vi "CIF Template UI.vi"() -> ()   [LabVIEW 2021, in "CIF Template UI.lvlib"]
uses:
  CIF Template UI.lvlib
  <vilib>/CIF Foundation/CIF Core/CIFUI/Typedef/Run Listen Button.ctl
  <vilib>/CIF Foundation/CIF Core/CIFUI/Typedef/Core UI References.ctl
  <vilib>/CIF Foundation/CIF Core/CIFUI/CIF_UI.lvclass/CIF_UI.ctl
  <vilib>/CIF Foundation/CIF Core/CIFUI/Utilities/Get Human Readable Error.vi
  <vilib>/CIF Foundation/CIF Utilities/Errors/Append Error Location.vi
  <vilib>/CIF Foundation/CIF Core/CIFUI/UI Element Update/Empty Tree by Reference.vi
  <vilib>/CIF Foundation/CIF Core/CIFUI/UI Element Update/Empty Table by Reference.vi
  <vilib>/CIF Foundation/CIF Core/CIFUI/UI Element Update/Initialize Manager Tab by Reference.vi
  <vilib>/CIF Foundation/CIF Utilities/Errors/Human Readable Error Message.vi
  <vilib>/CIF Foundation/CIF Core/CIFUI/CIF_UI.lvclass
  Grpc/Template_wrapper/Template_Wrapper.lvlib
  <vilib>/Utility/LVLibp/NI_PackedLibraryUtility.lvlib
panel:
  in  "Session Id":u64
  in  "EXIT":bool
  in  "Address with Port":string="192.168.1.160:12345"
  in  "Clear Local Error":bool
  out "Connected":bool
  in  "Unload":bool
  in  "Refresh Button":bool
  in  "Run Listen":T1
  in  "Connection":bool
  out "Local Error":string
  in  "Plugin Status":string[][](table)
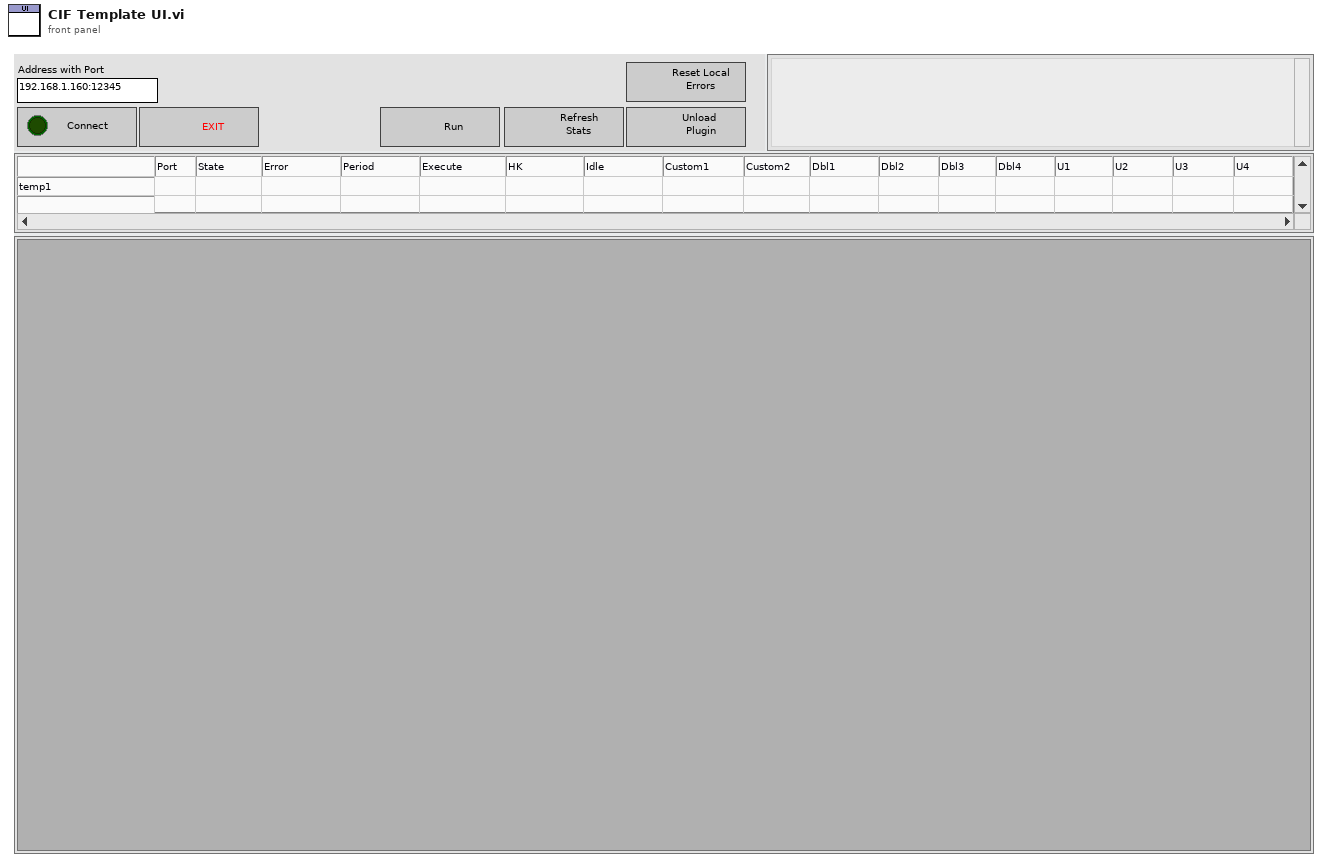
[diagram p1: front panel]
types:
  T1 = typedef "CIF_UI.lvclass/Run Listen Button.ctl" = bool
  T2 = typedef "CIF_UI.lvclass/Core UI References.ctl" = cluster{"Discovered Plugins":refnum<vi>, "Discovered Plugins Valid":bool, "Loaded Plugins":refnum<vi>, "Loaded Plugins Valid":bool, "Publisher Channels":refnum<vi>, "Publisher Channels Valid":bool, "Subscriber Channels":refnum<vi>, "Subscriber Channels Valid":bool, "Plugin Status":refnum<vi>, "Plugin Status Valid":bool, "Channel Connection":refnum<vi>, "Channel Connection Valid":bool, "New Plugin Load":refnum<vi>, "New Plugin Load Valid":bool, "Errors":refnum<vi>, "Errors Valid":bool, "Plugin to Abort":refnum<vi>, "Plugin to Abort Valid":bool, "Connection":refnum<vi>, "Connection Valid":bool, "Exit":refnum<vi>, "Exit Valid":bool, "Run Listen":refnum<vi>, "Run Listen Valid":bool, "CIF Manager Tab":refnum<vi>, "Manger Tab Valid":bool, "Clear Local Error":refnum<vi>, "Clear Local Error Valid":bool, "Local Error":refnum<vi>, "Local Error Valid":bool, "System Errors":refnum<vi>, "System Errors Valid":bool, "Plugin Selection":refnum<vi>, "Plugin Selection Valid":bool}
  T3 = typedef "CIF_InstrumentStudio Plugin SDK.lvlib/Event Registration Refnum.ctl" = refnum<event-registration>
  T4 = cluster{"Event Refnum":T3, "Event Registration Refnum":refnum<event-registration>}
  T5 = typedef "grpc-lvsupport-release.lvlib/grpcId.ctl" = u64
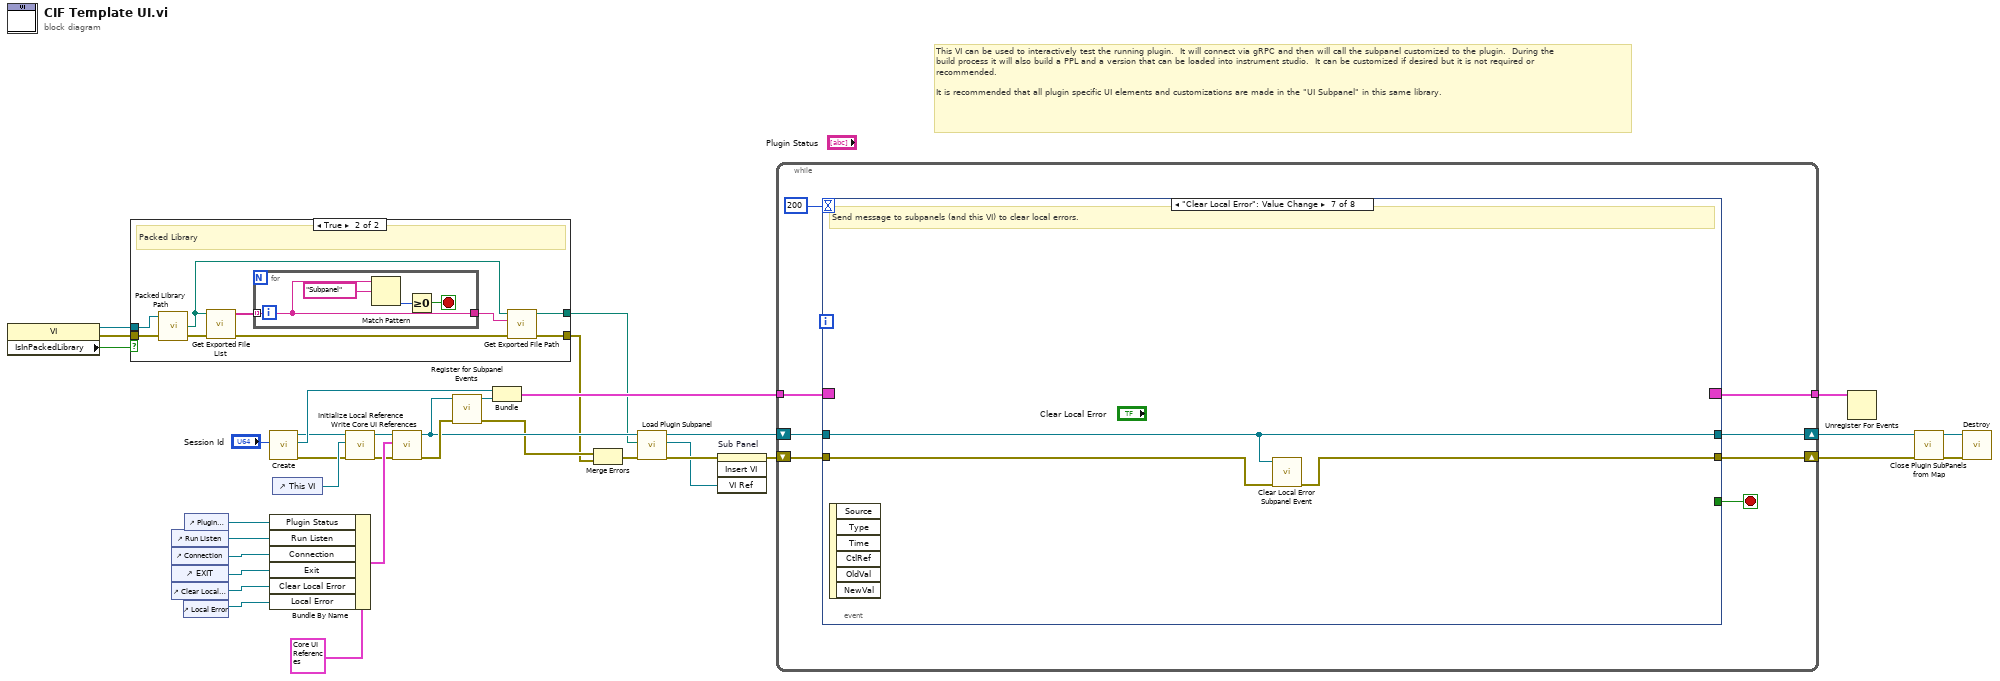
[diagram p0: block diagram]
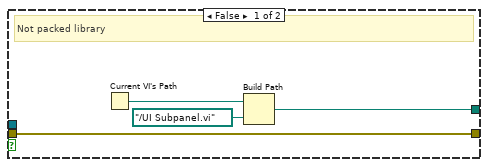
[diagram p2: hidden frame]
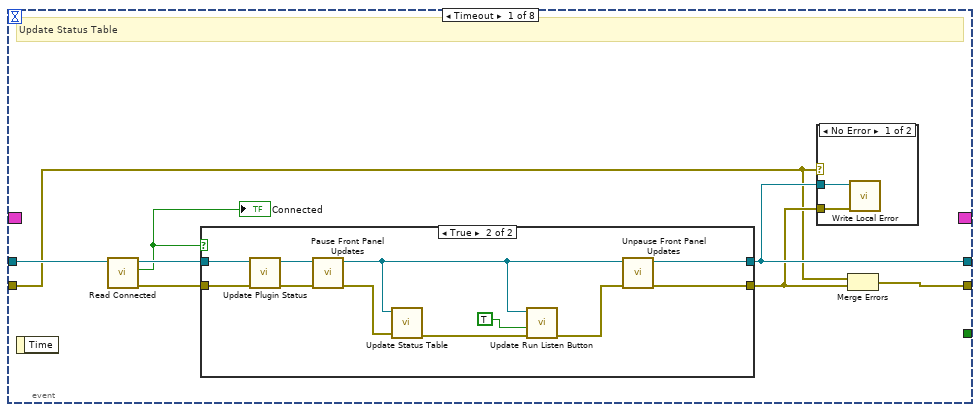
[diagram p3: hidden frame]
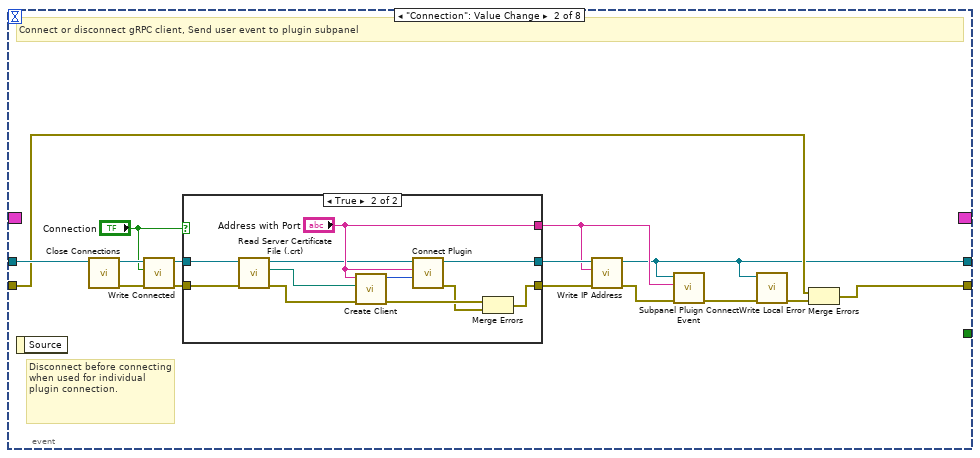
[diagram p6: hidden frame]
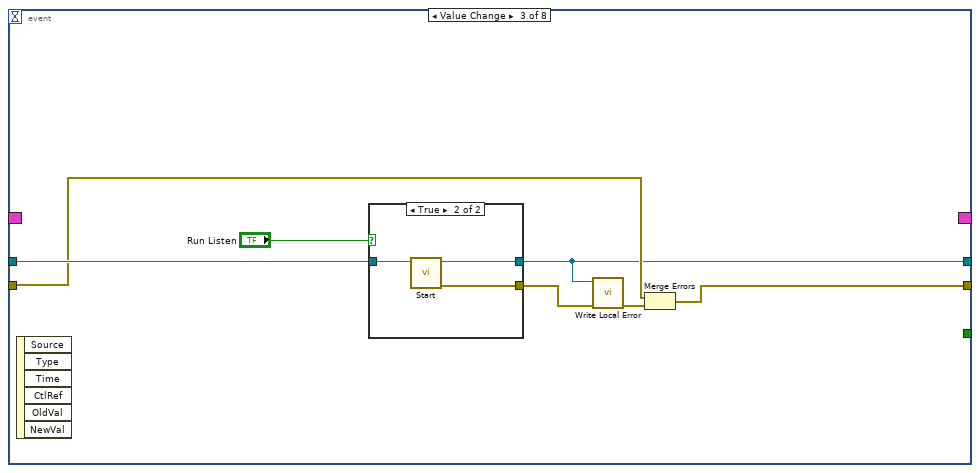
[diagram p8: hidden frame]
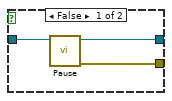
[diagram p9: hidden frame]
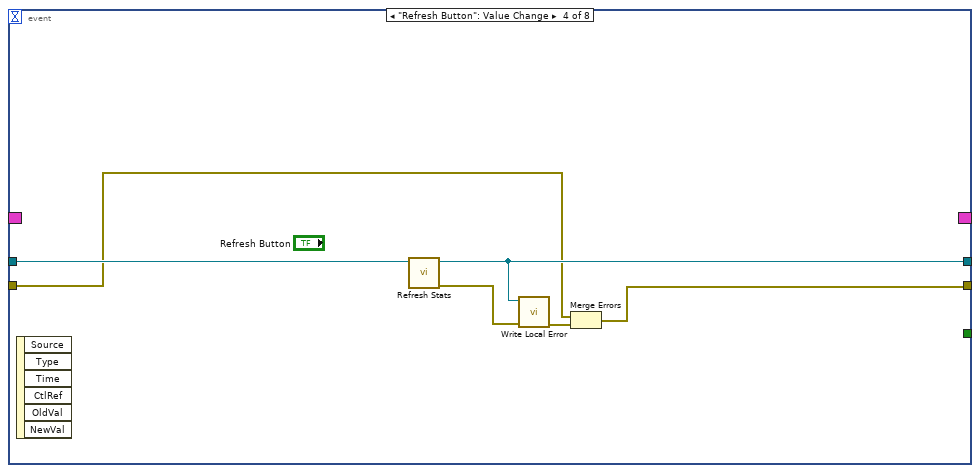
[diagram p10: hidden frame]
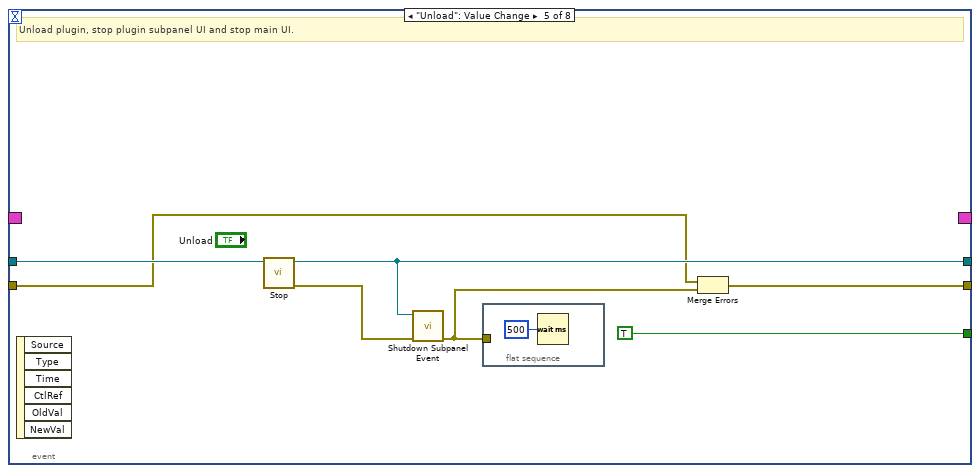
[diagram p11: hidden frame]
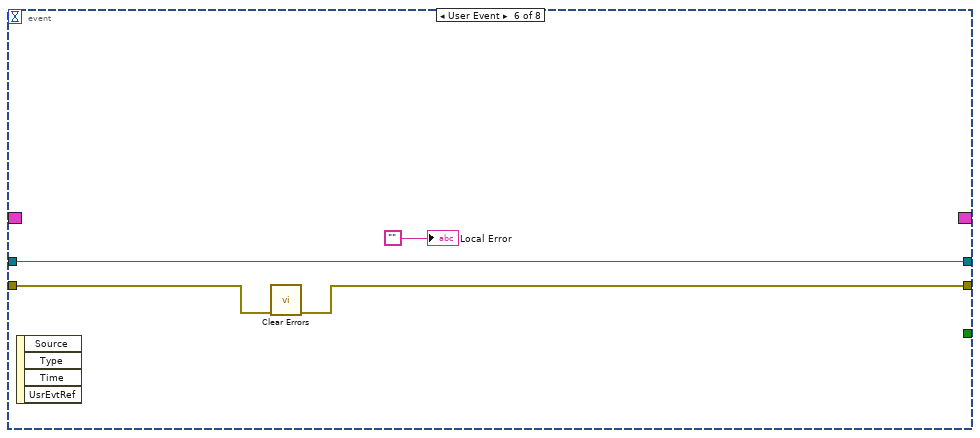
[diagram p12: hidden frame]
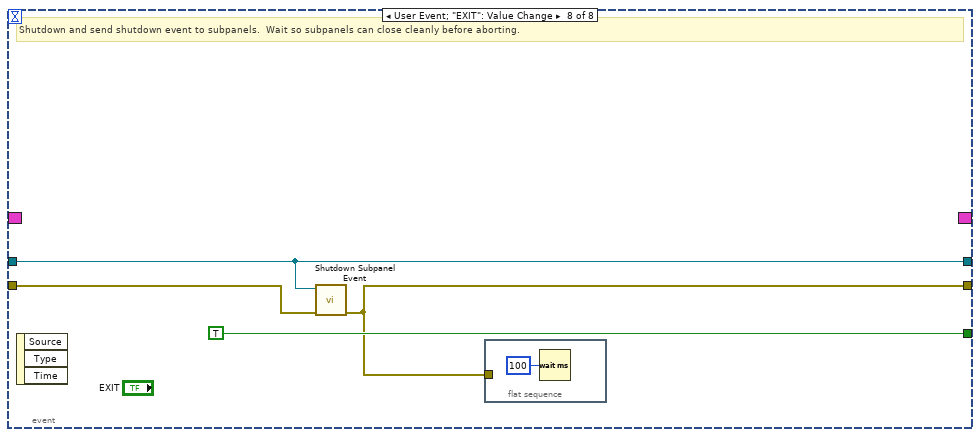
[diagram p13: hidden frame]
diagram:
  # "This VI can be used to interactively test the running plugin.  It will connect via gRPC and then will call the subpanel customized to the plugin.  During the build process it will also build a PPL and a version that can be loaded into instrument studio.  It can be customized if desired but it is not required or recommended.  \n\nIt is recommended that all plugin specific UI elements and customizations are made in the \"UI Subpanel\" in this same library."
  n1 = property class="VI"() -> (reference out=w8:refnum<vi>, error out=w7:errorcluster, "IsInPackedLibrary"=w9:bool)  [unwired: 2 in]
  n2 = case shown="True" w9 {
    tunnel: w8 -> [_ w48]
    tunnel: w7 -> [w36 w47]
    tunnel: [w39 w41] -> w6
    tunnel: [w36 w40] -> w3
    frame False {
      # "Not packed library"
      n3 = Current VI's Path() -> (path=w38:path)
      n4 = Build Path(base path=w38, name or relative path=path "../UI Subpanel.vi" ("Path")) -> (appended path=w39:path)
    }
    frame True {
      # "Packed Library"
      n5 = call <vilib>:"Packed Library Path.vi"("error in (no error)"=w47, "vi reference"=w48) -> ("error out"=w42:errorcluster, "packed library path"=w43:path)  [unwired: 1 in, 1 out]
      n6 = call <vilib>:"Get Exported File List.vi"("error in (no error)"=w42, "packed library path"=w43) -> ("error out"=w45:errorcluster, "qualified names"=w44:string[])  [unwired: 7 in, 1 out]
      n7 = for {
        tunnel: w44 -> [w49] mode=indexing
        tunnel: [w49] -> w46
        stop <- w51 stop-if-true
        n8 = Match Pattern(string=w49, regular expression="Subpanel") -> (offset past match=w52:i32)  [unwired: 1 in, 3 out]
        n9 = Greater Or Equal To 0?(x=w52) -> (x >= 0?=w51:bool)
      }
      n10 = call <vilib>:"Get Exported File Path.vi"("error in (no error)"=w45, "qualified name"=w46, "packed library path"=w43) -> ("error out"=w40:errorcluster, "path"=w41:path)  [unwired: 7 in]
    }
  }
  n11 = control-ref of="Run Listen"() -> (w29:refnum<vi>)
  n12 = control-ref of="Connection"() -> (w26:refnum<vi>)
  n13 = control-ref of="EXIT"() -> (w25:refnum<vi>)
  n14 = control-ref of="Clear Local Error"() -> (w24:refnum<vi>)
  n15 = control-ref of="Local Error"() -> (w23:refnum<vi>)
  n16 = control-ref of="Plugin Status"() -> (w33:refnum<vi>)
  n17 = call <vilib>:"Create.vi"("Session Id"="Session Id") -> ("error out"=w20:errorcluster, "Event Refnum"=w27:T3, "CIF_UI out"=w21:refnum<class "CIF_UI.lvclass">)  [unwired: 8 in]
  n18 = Bundle By Name(cluster=T2 {"Discovered Plugins"=refnum, "Discovered Plugins Valid"=FALSE, "Loaded Plugins"=refnum, "Loaded Plugins Valid"=FALSE, "Publisher Channels"=refnum, "Publisher Channels Valid"=FALSE, "Subscriber Channels"=refnum, "Subscriber Channels Valid"=FALSE, "Plugin Status"=refnum, "Plugin Status Valid"=FALSE, "Channel Connection"=refnum, "Channel Connection Valid"=FALSE, "New Plugin Load"=refnum, "New Plugin Load Valid"=FALSE, "Errors"=refnum, "Errors Valid"=FALSE, "Plugin to Abort"=refnum, "Plugin to Abort Valid"=FALSE, "Connection"=refnum, "Connection Valid"=FALSE, "Exit"=refnum, "Exit Valid"=FALSE, "Run Listen"=refnum, "Run Listen Valid"=FALSE, "CIF Manager Tab"=refnum, "Manger Tab Valid"=FALSE, "Clear Local Error"=refnum, "Clear Local Error Valid"=FALSE, "Local Error"=refnum, "Local Error Valid"=FALSE, "System Errors"=refnum, "System Errors Valid"=FALSE, "Plugin Selection"=refnum, "Plugin Selection Valid"=FALSE} ("UI References"), "Plugin Status"=w33, "Run Listen"=w29, "Connection"=w26, "Exit"=w25, "Clear Local Error"=w24, "Local Error"=w23) -> (w34:T2)
  n19 = control-ref of="This VI"() -> (w32:refnum<vi>)
  n20 = call <vilib>:"Initialize Local Reference.vi"("error in (no error)"=w20, "This VI"=w32, "CIF_UI in"=w21) -> ("error out"=w30:errorcluster, "CIF_UI out"=w31:refnum<class "CIF_UI.lvclass">)  [unwired: 7 in]
  n21 = call <vilib>:"Write Core UI References.vi"("error in (no error)"=w30, "UI References"=w34, "CIF_UI in"=w31) -> ("error out"=w19:errorcluster, "CIF_UI out"=w17:refnum<class "CIF_UI.lvclass">)  [unwired: 7 in]
  n22 = call <vilib>:"Register for Subpanel Events.vi"("error in (no error)"=w19, "CIF_UI in"=w17) -> ("error out"=w5:errorcluster, "Event Registration Refnum"=w28:refnum<event-registration>)  [unwired: 8 in]
  n23 = Bundle("Event Refnum"=w27, "Event Registration Refnum"=w28) -> (w22:T4)  [unwired: 1 in]
  n24 = Merge Errors(w5, w3) -> (w4:errorcluster)
  n25 = call <vilib>:"Load Plugin Subpanel.vi"("error in (no error)"=w4, "Path"=w6, "CIF_UI in"=w17) -> ("error out"=w15:errorcluster, "VI Reference"=w13:refnum<vi>, "CIF_UI out"=w16:refnum<class "CIF_UI.lvclass">)  [unwired: 6 in]
  n26 = invoke on="Sub Panel" class="SubPnl" method="Insert VI"(error in=w15, "VI Ref"=w13) -> (error out=w14:errorcluster)  [unwired: 2 in, 3 out]
  n27 = while {
    shift-right: [w55] -> w12
    shift-left: w16 -> [w58]
    shift-right: [w56] -> w1
    shift-left: w14 -> [w57]
    tunnel: w22 -> [w54]
    tunnel: [w53] -> w18
    stop <- w59 stop-if-true
    n28 = event shown="[6] \"Clear Local Error\": Value Change" {
      selector: w54 -> [_ _ _ _ _ _ _ _]
      dyn-events: [_ _ _ _ _ _ _ _] -> w53
      timeout: 200 -> [_ _ _ _ _ _ _ _]
      tunnel: [_ _ _ _ TRUE _ _ TRUE] -> w59
      tunnel: w58 -> [w66 w98 w118 w130 w137 w140 w143 w148]
      tunnel: w57 -> [w61 w86 w114 w125 w132 w142 w145 w147]
      tunnel: [w64 w85 w113 w126 w131 w141 w144 w146] -> w56
      tunnel: [w63 w84 w112 w127 w135 w140 w143 w148] -> w55
      event Timeout {
        # "Update Status Table"
        n29 = event-data() -> ()  [unwired: 1 in, 1 out]
        n30 = call <vilib>:"Read Connected.vi"("CIF_UI in"=w66) -> ("error out"=w67:errorcluster, "Connected"=w65:bool, "CIF_UI out"=w68:refnum<class "CIF_UI.lvclass">)  [unwired: 8 in]
        "Connected" <- w65
        n31 = case shown="True" w65 {
          tunnel: w67 -> [w71 w81]
          tunnel: [w71 w83] -> w62
          tunnel: w68 -> [w72 w80]
          tunnel: [w72 w82] -> w63
          frame False {
          }
          frame True {
            n32 = call <vilib>:"Update Plugin Status.vi"("error in (no error)"=w81, "CIF_UI in"=w80) -> ("error out"=w77:errorcluster, "CIF_UI out"=w79:refnum<class "CIF_UI.lvclass">)  [unwired: 8 in]
            n33 = call <vilib>:"Pause Front Panel Updates.vi"("error in (no error)"=w77, "CIF_UI in"=w79) -> ("error out"=w78:errorcluster, "CIF_UI out"=w74:refnum<class "CIF_UI.lvclass">)  [unwired: 8 in]
            n34 = call <vilib>:"Update Status Table.vi"("error in (no error)"=w78, "CIFManager_UI in"=w74) -> ("error out"=w76:errorcluster)  [unwired: 9 in]
            n35 = call <vilib>:"Update Run Listen Button.vi"("error in (no error)"=w76, "Use First Entry"=TRUE, "CIFManager_UI in"=w74) -> ("error out"=w75:errorcluster)  [unwired: 8 in]
            n36 = call <vilib>:"Unpause Front Panel Updates.vi"("error in (no error)"=w75, "CIF_UI in"=w74) -> ("error out"=w83:errorcluster, "CIF_UI out"=w82:refnum<class "CIF_UI.lvclass">)  [unwired: 8 in]
          }
        }
        n37 = case shown="No Error" w61 {
          tunnel: w62 -> [w70 _]
          tunnel: w63 -> [w69 _]
          frame No Error {
            n38 = call <vilib>:"Write Local Error.vi"("error in (no error)"=w70, "CIF_UI in"=w69) -> ()  [unwired: 9 in, 1 out]
          }
          frame Error {
          }
        }
        n39 = Merge Errors(w61, w62) -> (w64:errorcluster)
      }
      event "Connection": Value Change {
        # "Disconnect before connecting when used for individual plugin connection."
        # "Connect or disconnect gRPC client, Send user event to plugin subpanel"
        n40 = event-data() -> ()  [unwired: 1 in, 1 out]
        n41 = call <vilib>:"Close Connections.vi"("CIF_UI in"=w98) -> ("error out"=w96:errorcluster, "CIF_UI out"=w97:refnum<class "CIF_UI.lvclass">)  [unwired: 9 in]
        n42 = call <vilib>:"Write Connected.vi"("error in (no error)"=w96, "Connected"="Connection", "CIF_UI in"=w97) -> ("error out"=w93:errorcluster, "CIF_UI out"=w95:refnum<class "CIF_UI.lvclass">)  [unwired: 7 in]
        n43 = case shown="True" "Connection" {
          tunnel: [w100 w107] -> w92
          tunnel: [w99 w111] -> w91
          tunnel: w93 -> [w99 w104]
          tunnel: w95 -> [w100 w105]
          tunnel: [_ "Address with Port"] -> w89
          frame False {
          }
          frame True {
            n44 = call <vilib>:"Read Server Certificate File (.crt).vi"("error in (no error)"=w104, "CIF_UI in"=w105) -> ("error out"=w103:errorcluster, "Server Certificate File (.crt)"=w102:path, "CIF_UI out"=w101:refnum<class "CIF_UI.lvclass">)  [unwired: 7 in]
            n45 = call "Create Client.vi"("error in"=w103, "Server Certificate File (.crt)"=w102, "address"="Address with Port") -> ("error out"=w109:errorcluster, "gRPC ID Out"=w110:T5)  [unwired: 7 in]
            n46 = call <vilib>:"Connect Plugin.vi"("gRPC ID"=w110, "Address"="Address with Port", "CIF_UI in"=w101) -> ("error out"=w108:errorcluster, "CIF_UI out"=w107:refnum<class "CIF_UI.lvclass">)  [unwired: 7 in]
            n47 = Merge Errors(w109, w108) -> (w111:errorcluster)
          }
        }
        n48 = call <vilib>:"Write IP Address.vi"("error in (no error)"=w91, "IP Address"=w89, "CIF_UI in"=w92) -> ("error out"=w90:errorcluster, "CIF_UI out"=w84:refnum<class "CIF_UI.lvclass">)  [unwired: 7 in]
        n49 = call <vilib>:"Subpanel Pluign Connect Event.vi"("error in (no error)"=w90, "Address and Port"=w89, "CIF_UI in"=w84) -> ("error out"=w87:errorcluster)  [unwired: 8 in]
        n50 = call <vilib>:"Write Local Error.vi"("error in (no error)"=w87, "CIF_UI in"=w84) -> ("error out"=w88:errorcluster)  [unwired: 9 in]
        n51 = Merge Errors(w86, w88) -> (w85:errorcluster)
      }
      event Value Change {
        n52 = event-data() -> ()  [unwired: 1 in, 6 out]
        n53 = case shown="True" "Run Listen" {
          tunnel: w118 -> [w121 w124]
          tunnel: [w119 w123] -> w112
          tunnel: [w120 w122] -> w115
          frame False {
            n54 = call <vilib>:"Pause.vi"("CIF_Plugin_UI in"=w121) -> ("error out"=w120:errorcluster, "CIF_Plugin_UI out"=w119:refnum<class "CIF_UI.lvclass">)  [unwired: 8 in, 1 out]
          }
          frame True {
            n55 = call <vilib>:"Start.vi"("CIF_Plugin_UI in"=w124) -> ("error out"=w122:errorcluster, "CIF_Plugin_UI out"=w123:refnum<class "CIF_UI.lvclass">)  [unwired: 8 in, 1 out]
          }
        }
        n56 = call <vilib>:"Write Local Error.vi"("error in (no error)"=w115, "CIF_UI in"=w112) -> ("error out"=w116:errorcluster)  [unwired: 9 in]
        n57 = Merge Errors(w114, w116) -> (w113:errorcluster)
      }
      event "Refresh Button": Value Change {
        n58 = event-data() -> ()  [unwired: 1 in, 6 out]
        n59 = call <vilib>:"Refresh Stats.vi"("CIF_Plugin_UI in"=w130) -> ("error out"=w128:errorcluster, "CIF_Plugin_UI out"=w127:refnum<class "CIF_UI.lvclass">)  [unwired: 8 in, 1 out]
        n60 = call <vilib>:"Write Local Error.vi"("error in (no error)"=w128, "CIF_UI in"=w127) -> ("error out"=w129:errorcluster)  [unwired: 9 in]
        n61 = Merge Errors(w125, w129) -> (w126:errorcluster)
      }
      event "Unload": Value Change {
        # "Unload plugin, stop plugin subpanel UI and stop main UI."
        n62 = event-data() -> ()  [unwired: 1 in, 6 out]
        n63 = call <vilib>:"Stop.vi"("CIF_Plugin_UI in"=w137) -> ("error out"=w136:errorcluster, "CIF_Plugin_UI out"=w135:refnum<class "CIF_UI.lvclass">)  [unwired: 8 in, 1 out]
        n64 = call <vilib>:"Shutdown Subpanel Event.vi"("error in (no error)"=w136, "CIF_UI in"=w135) -> ("error out"=w133:errorcluster)  [unwired: 9 in]
        n65 = flat-sequence {
          tunnel: w133 -> [_]
          frame #0 {
            n66 = Wait (ms)(milliseconds to wait=u32 500) -> ()  [unwired: 1 out]
          }
        }
        n67 = Merge Errors(w132, w133) -> (w131:errorcluster)
      }
      event User Event {
        n68 = event-data() -> ()  [unwired: 1 in, 4 out]
        n69 = call <vilib>:"Clear Errors.vi"("error in (no error)"=w142) -> ("error out"=w141:errorcluster)  [unwired: 5 in, 1 out]
        "Local Error" <- ""
      }
      event "Clear Local Error": Value Change {
        # "Send message to subpanels (and this VI) to clear local errors."
        n70 = event-data() -> ()  [unwired: 1 in, 6 out]
        n71 = call <vilib>:"Clear Local Error Subpanel Event.vi"("error in (no error)"=w145, "CIF_UI in"=w143) -> ("error out"=w144:errorcluster)  [unwired: 9 in]
      }
      event User Event; "EXIT": Value Change {
        # "Shutdown and send shutdown event to subpanels.  Wait so subpanels can close cleanly before aborting."
        n72 = event-data() -> ()  [unwired: 1 in, 3 out]
        n73 = call <vilib>:"Shutdown Subpanel Event.vi"("error in (no error)"=w147, "CIF_UI in"=w148) -> ("error out"=w146:errorcluster)  [unwired: 9 in]
        n74 = flat-sequence {
          tunnel: w146 -> [_]
          frame #0 {
            n75 = Wait (ms)(milliseconds to wait=u32 100) -> ()  [unwired: 1 out]
          }
        }
      }
    }
  }
  n76 = Unregister For Events(event registration refnum=w18) -> ()  [unwired: 1 in, 1 out]
  n77 = call <vilib>:"Close Plugin SubPanels from Map.vi"("error in (no error)"=w1, "CIF_UI in"=w12) -> ("error out"=w11:errorcluster, "CIF_UI out"=w10:refnum<class "CIF_UI.lvclass">)  [unwired: 8 in]
  n78 = call <vilib>:"Destroy.vi"("error in (no error)"=w11, "CIF_UI in"=w10) -> ()  [unwired: 8 in, 2 out]
